vi "Template Get All sStyle.vi"(8 "error in (no error)":errorcluster, 10 "sStyle (\"\")":string, 11 "Connection Refnum":T1) -> (0 "error out":errorcluster, 2 "Templates":T2[](array[typedef]), 3 "Connection Refnum":T1, 4 "Data Present":bool)   [LabVIEW 2011]
uses:
  Template Record.ctl
  SI.LIB/ODBC/SQL Controls/Connection Refnum.ctl
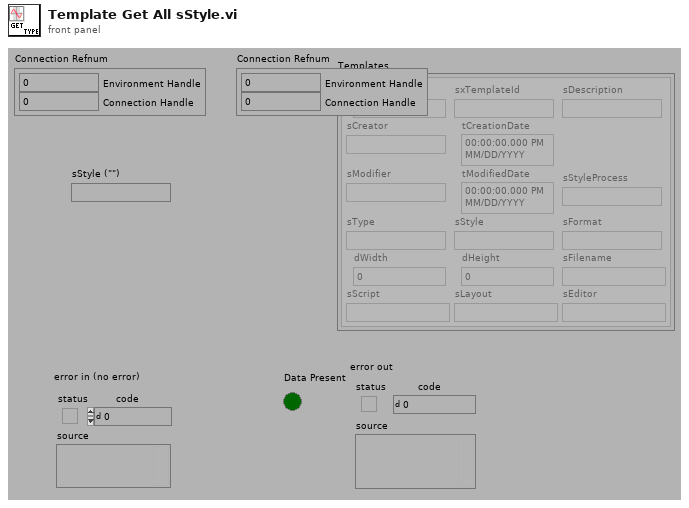
[diagram p1: front panel]
types:
  T1 = typedef "Connection Refnum.ctl" = cluster{"Environment Handle":i32, "Connection Handle":i32}
  T2 = typedef "Template Record.ctl" = cluster{"ixTemplate":i32, "sxTemplateId":string, "sDescription":string, "sCreator":string, "tCreationDate":timestamp, "sModifier":string, "tModifiedDate":timestamp, "sType":string, "sStyle":string, "sFormat":string, "dWidth":dbl, "dHeight":dbl, "sFilename":string, "sScript":string, "sLayout":string, "sEditor":string, "sStyleProcess":string}
  T3 = typedef "Statement Refnum.ctl" = cluster{"Statement Handle":i32, "Parameter Number":u16}
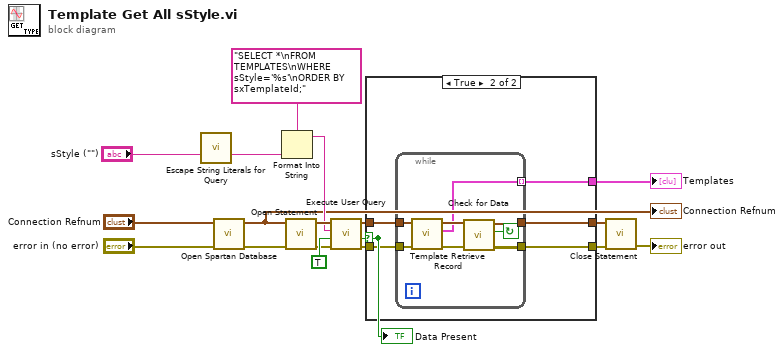
[diagram p0: block diagram]
diagram:
  n1 = call "Escape String Literals for Query.vi"("String"="sStyle (\"\")") -> ("escaped String"=w5:string)  [unwired: 1 in, 13 out]
  n2 = call "Open Spartan Database.vi"("error in (no error)"="error in (no error)", "DB Path (empty - use default)"="Connection Refnum") -> ("error out"=w10:errorcluster, "Connection Refnum"=w2:T1)  [unwired: 8 out]
  "Connection Refnum" <- w2
  n3 = Format Into String(format string="SELECT *\nFROM TEMPLATES\nWHERE sStyle='%s'\nORDER BY sxTemplateId;" ("Query Name"), w5) -> (resulting string=w7:string)  [unwired: 2 in, 1 out]
  n4 = call "Open Statement.vi"("error in (no error)"=w10, "Connection Refnum"=w2) -> ("error out"=w12:errorcluster, "Statement Refnum"=w13:T3)  [unwired: 4 out]
  n5 = call "Execute User Query.vi"("error in (no error)"=w12, "Return Data? (f)"=TRUE, "User Query"=w7, "Statement Refnum"=w13) -> ("error out"=w18:errorcluster, "Data Present?"=w9:bool, "Statement Refnum"=w17:T3)  [unwired: 1 out]
  "Data Present" <- w9
  n6 = case shown="True" w9 {
    tunnel: w18 -> [w19 w24]
    tunnel: w17 -> [w20 w25]
    tunnel: [w19 w22] -> w14
    tunnel: [w20 w23] -> w15
    tunnel: [_ w21] -> w1
    frame False {
    }
    frame True {
      n7 = while {
        tunnel: w25 -> [w32]
        tunnel: w24 -> [w31]
        tunnel: [w29] -> w23
        tunnel: [w27] -> w22
        tunnel: [w26] -> w21 mode=indexing
        stop <- w33 continue-if-true
        n8 = call "Template Retrieve Record.vi"("error in (no error)"=w31, "Statement Refnum"=w32) -> ("error out"=w28:errorcluster, "Template Record"=w26:T2, "Statement Refnum"=w30:T3)  [unwired: 7 out]
        n9 = call "Check for Data.vi"("error in (no error)"=w28, "Statement Refnum"=w30) -> ("error out"=w27:errorcluster, "Data Present?"=w33:bool, "Statement Refnum"=w29:T3)  [unwired: 3 out]
      }
    }
  }
  "Templates" <- w1
  n10 = call "Close Statement.vi"("error in (no error)"=w14, "Statement Refnum"=w15) -> ("error out"=→"error out":errorcluster)  [unwired: 5 out]
